vi "AMC Create Message.vi"(6 "Attributes":T1, 8 "Value":string, 9 "Name":string) -> (1 "Message":T2)   [LabVIEW 2009]
doc: "This VI is used for compatibility with previous versions of the AMC library. Use the AMC VIs located in the <b>Data Communication >> Asynchronous Message Communication</b> palette."
uses:
  Message.ctl
  <vilib>/NI/Tools/Keyed Array/KeyedArray.ctl
  Create Single Message.vi
  AMC.lvlib
  <vilib>/NI/Tools/Keyed Array/Tools_KeyedArray.lvlib
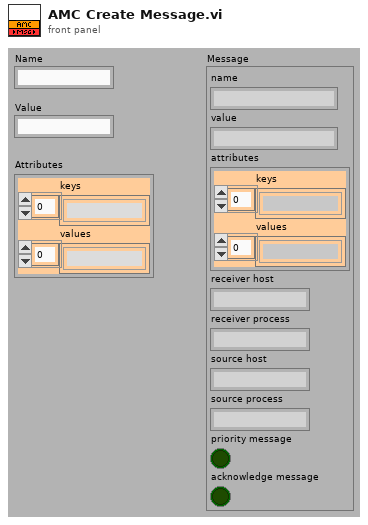
[diagram p1: front panel]
types:
  T1 = typedef "Tools_KeyedArray.lvlib/KeyedArray.ctl" = cluster{"keys":string[], "values":string[]}
  T2 = typedef "AMC.lvlib/Message.ctl" = cluster{"name":string, "value":string, "attributes":T1, "receiver host":string, "receiver process":string, "source host":string, "source process":string, "priority message":bool, "acknowledge message":bool}
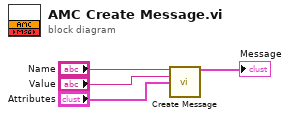
[diagram p0: block diagram]
diagram:
  n1 = call-poly "Create Message.vi"("name"="Name", "value"="Value", "attributes"="Attributes") -> ("message"=→"Message":T2)  [unwired: 11 in, 1 out]
